vi "ModbusComap.vi"(0 "address":string="192.168.1.205", 1 "port (502)":u16=502, 2 "Unit ID":u8, 3 "Error In":errorcluster) -> (7 "Gen Data":T1 {"TotalFuel(L)" format="%.2f"; "FuelRate(L/H)" format="%.2f"; "ApparentPower(VA)" format="%.2f"; "BattVoltage(V)" format="%.2f"; "Freq(Hz)" format="%.2f"; "RunHours(hr)" format="%.2f"; "PowerFactor" format="%.2f"; "ReactivePower(VAR)" format="%.2f"; "ActivePower(W)" format="%.2f"}, 10 "Error Out":errorcluster)   [LabVIEW 2014]
uses:
  Controls/Gen Data.ctl
  Controls/ModbusState.ctl
  <vilib>/Modbus/master/Modbus Master.lvclass
  <vilib>/Modbus/subvis/Modbus API/Modbus API.lvclass/Modbus API.ctl
  <vilib>/Modbus/subvis/Transmission Data Unit (ADU)/Transmission Data Unit/Transmission Data Unit.lvclass/Transmission Data Unit.ctl
  <vilib>/Modbus/master/Data Access/Unit ID/Set Unit ID Property.vi
  <vilib>/Modbus/subvis/Transmission Data Unit (ADU)/Transmission Data Unit/Data Access/Unit ID/Write Unit ID.vi
  <vilib>/Modbus/subvis/Modbus API/Read Transmission Data Unit.vi
  <vilib>/Modbus/subvis/Modbus API/Write Transmission Data Unit.vi
  <vilib>/Modbus/master/Create Master Instance (TCP).vi
  <vilib>/Modbus/subvis/Transmission Data Unit (ADU)/Transmission Data Unit/Transmission Data Unit.lvclass
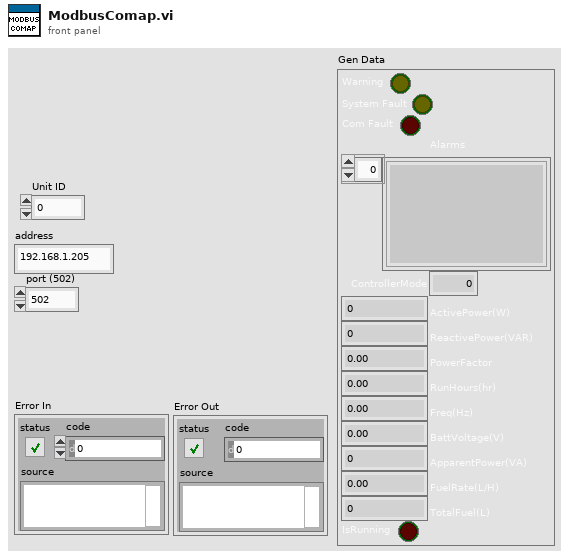
[diagram p1: front panel]
types:
  T1 = typedef "Gen Data.ctl" = cluster{"Warning":bool, "System Fault":bool, "Com Fault":bool, "Alarms":string[], "ControllerMode":u16, "ActivePower(W)":i32, "ReactivePower(VAR)":i32, "PowerFactor":dbl, "RunHours(hr)":dbl, "Freq(Hz)":dbl, "BattVoltage(V)":dbl, "ApparentPower(VA)":i32, "FuelRate(L/H)":dbl, "TotalFuel(L)":u32, "IsRunning":bool}
  T2 = typedef "ModbusState.ctl" = enum16{"Connect", "Disconnect", "Set Basic Objects", "Get Basic Objects", "Read", "Write", "Read/Write"}
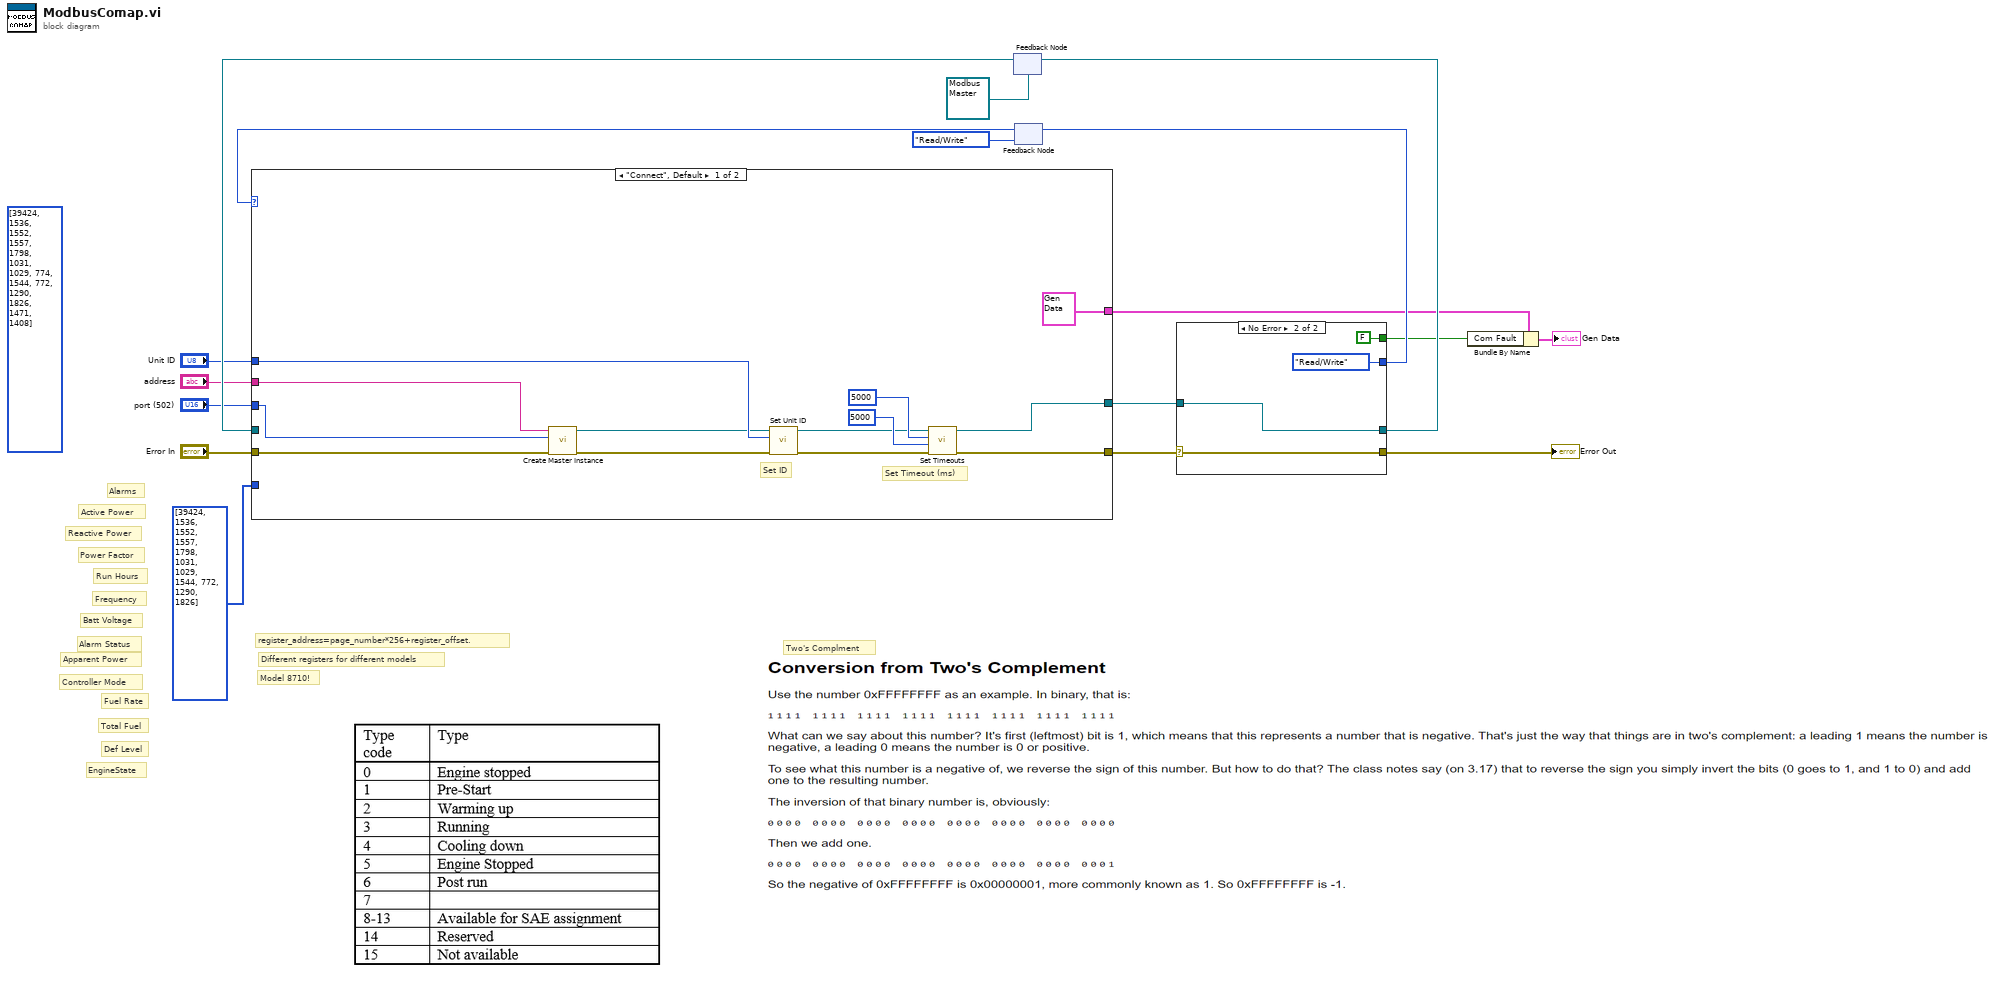
[diagram p0: block diagram]
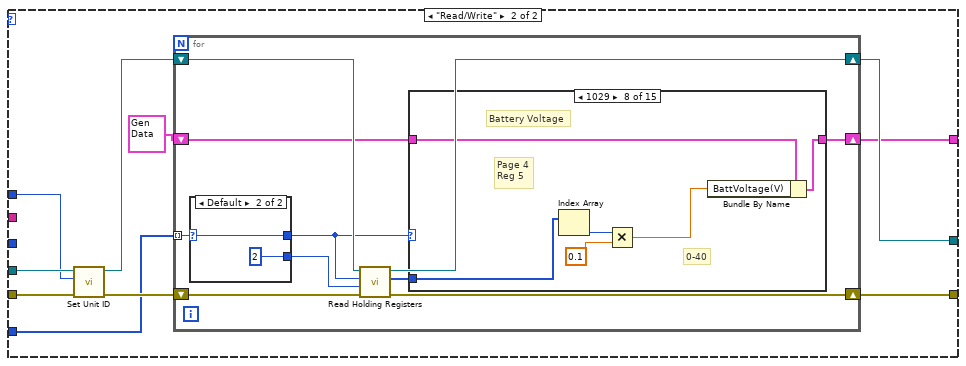
[diagram p2: hidden frame]
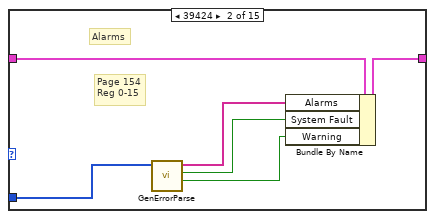
[diagram p4: hidden frame]
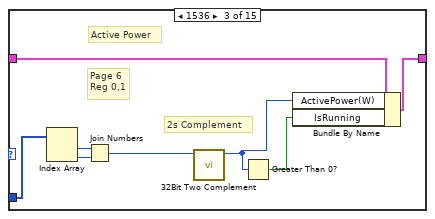
[diagram p5: hidden frame]
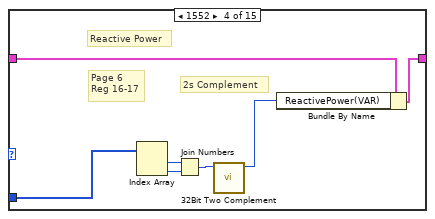
[diagram p6: hidden frame]
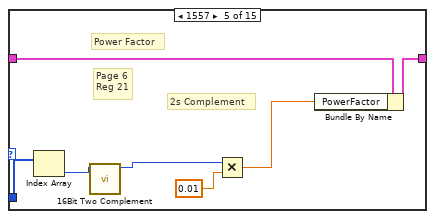
[diagram p7: hidden frame]
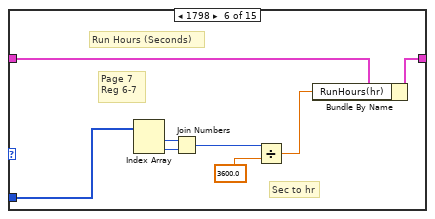
[diagram p8: hidden frame]
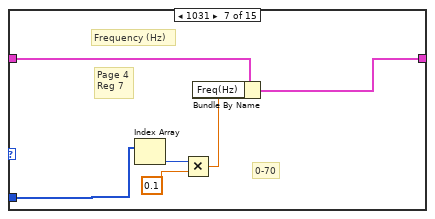
[diagram p9: hidden frame]
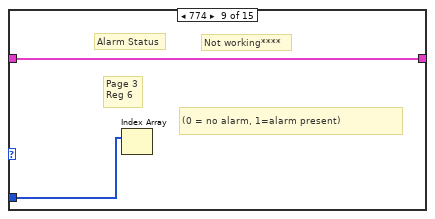
[diagram p10: hidden frame]
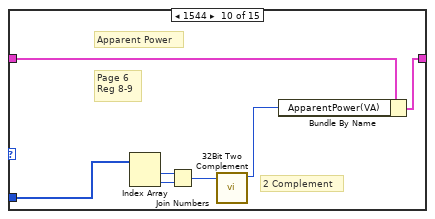
[diagram p11: hidden frame]
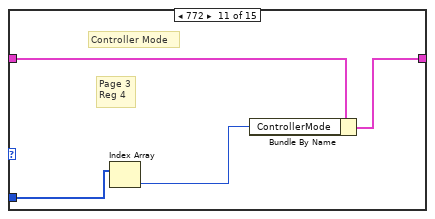
[diagram p12: hidden frame]
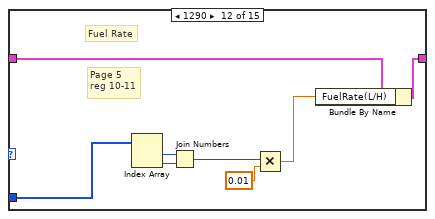
[diagram p13: hidden frame]
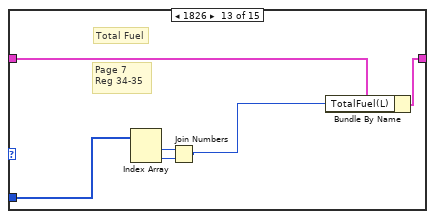
[diagram p14: hidden frame]
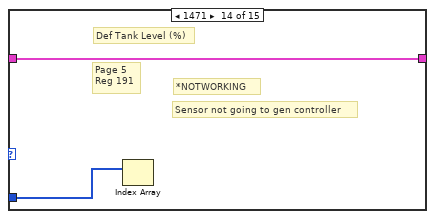
[diagram p15: hidden frame]
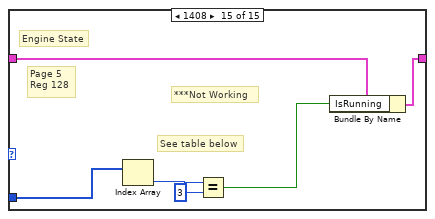
[diagram p16: hidden frame]
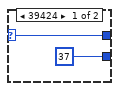
[diagram p17: hidden frame]
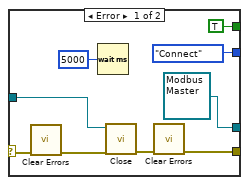
[diagram p18: hidden frame]
diagram:
  (unwired) u16[] [39424, 1536, 1552, 1557, 1798, 1031, 1029, 774, 1544, 772, 1290, 1826, 1471, 1408] ("subarray")
  # "EngineState"
  # "Two's Complment"
  # "Different registers for different models"
  # "Model 8710!"
  # "Def Level"
  # "Alarm Status"
  # "Controller Mode"
  # "register_address=page_number*256+register_offset."
  # "Total Fuel"
  # "Fuel Rate"
  # "Apparent Power"
  # "Run Hours"
  # "Power Factor"
  # "Reactive Power"
  # "Active Power"
  # "Alarms"
  # "Batt Voltage"
  # "Frequency"
  n1 = feedback #1(refnum<class "Modbus Master.lvclass"> refnum ("Modbus master out")) -> (w13:refnum<class "Modbus Master.lvclass">)
  n2 = feedback #2(ModbusState."Read/Write" ("Modbus State In")) -> (w16:T2)
  n3 = case shown="\"Connect\", Default" w16 {
    tunnel: "Error In" -> [w30 w40]
    tunnel: w13 -> [_ w39]
    tunnel: [w19 w35] -> w10
    tunnel: [w18 w36] -> w8
    tunnel: [T1 {"Warning"=FALSE, "System Fault"=FALSE, "Com Fault"=FALSE, "Alarms"=[], "ControllerMode"=0, "ActivePower(W)"=0, "ReactivePower(VAR)"=0, "PowerFactor"=0.0, "RunHours(hr)"=0.0, "Freq(Hz)"=0.0, "BattVoltage(V)"=0.0, "ApparentPower(VA)"=0, "FuelRate(L/H)"=0.0, "TotalFuel(L)"=0, "IsRunning"=FALSE} ("Gen Data") w31] -> w2
    tunnel: "address" -> [w27 _]
    tunnel: "port (502)" -> [w26 _]
    tunnel: "Unit ID" -> [w21 w38]
    tunnel: u16[] [39424, 1536, 1552, 1557, 1798, 1031, 1029, 1544, 772, 1290, 1826] ("subarray") -> [_ w32]
    frame "Connect", Default {
      # "Set Timeout (ms)"
      # "Set ID"
      n4 = call-poly <vilib>:"Create Master Instance.vi"("error in (no error)"=w30, "port (502)"=w26, "address"=w27) -> ("error out"=w24:errorcluster, "TCP master instance"=w20:refnum<class "Modbus Master.lvclass">)  [unwired: 7 in]
      n5 = call <vilib>:"Set Unit ID.vi"("error in (no error)"=w24, "unit ID"=w21, "Modbus master in"=w20) -> ("error out"=w23:errorcluster, "Modbus master out"=w22:refnum<class "Modbus Master.lvclass">)  [unwired: 7 in]
      n6 = call <vilib>:"Set Timeouts.vi"("error in (no error)"=w23, "write operation timeout (ms)"=5000 ("write operation timeout"), "read operation timeout (ms)"=5000 ("read operation timeout"), "Modbus master in"=w22) -> ("error out"=w19:errorcluster, "Modbus master out"=w18:refnum<class "Modbus Master.lvclass">)  [unwired: 6 in]
    }
    frame "Read/Write" {
      n7 = call <vilib>:"Set Unit ID.vi"("error in (no error)"=w40, "unit ID"=w38, "Modbus master in"=w39) -> ("error out"=w33:errorcluster, "Modbus master out"=w34:refnum<class "Modbus Master.lvclass">)  [unwired: 7 in]
      n8 = for {
        tunnel: w32 -> [w50] mode=indexing
        shift-right: [w41] -> w35
        shift-left: w33 -> [w48]
        shift-right: [w46] -> w36
        shift-left: w34 -> [w47]
        shift-right: [w42] -> w31
        shift-left: T1 {"Warning"=FALSE, "System Fault"=FALSE, "Com Fault"=FALSE, "Alarms"=[], "ControllerMode"=0, "ActivePower(W)"=0, "ReactivePower(VAR)"=0, "PowerFactor"=0.0, "RunHours(hr)"=0.0, "Freq(Hz)"=0.0, "BattVoltage(V)"=0.0, "ApparentPower(VA)"=0, "FuelRate(L/H)"=0.0, "TotalFuel(L)"=0, "IsRunning"=FALSE} ("Gen Data") -> [w43]
        n9 = case shown="Default" w50 {
          selector: w50 -> [w135 w138]
          tunnel: [w135 w138] -> w45
          tunnel: [u16 37 ("number of inputs") u16 2 ("number of inputs")] -> w49
          frame 39424 {
          }
          frame Default {
          }
        }
        n10 = call-dynamic "Read Holding Registers.vi"("error in (no error)"=w48, "number of holding registers"=w49, "starting address"=w45, "Modbus master in"=w47) -> ("error out"=w41:errorcluster, "register values"=w44:u16[], "Modbus master out"=w46:refnum<class "Modbus Master.lvclass">)  [unwired: 5 in]
        n11 = case shown="1029" w45 {
          tunnel: w44 -> [_ w55 w63 w68 w77 w83 w91 w95 w101 w104 w112 w117 w122 w128 w132]
          tunnel: w43 -> [w51 w57 w65 w72 w79 w87 w93 w99 w100 w108 w111 w120 w126 w127 w134]
          tunnel: [w51 w56 w64 w71 w78 w86 w92 w98 w100 w107 w110 w119 w125 w127 w133] -> w42
          frame Default {
          }
          frame 39424 {
            # "Page 154\nReg 0-15"
            # "Alarms"
            n12 = call "GenErrorParse.vi"("register values"=w55) -> ("Warning"=w52:bool, "SystemFault"=w53:bool, "Alarms"=w54:string[])  [unwired: 8 in]
            n13 = Bundle By Name(cluster=w57, "Alarms"=w54, "System Fault"=w53, "Warning"=w52) -> (w56:T1)
          }
          frame 1536 {
            # "2s Complement"
            # "Page 6\nReg 0,1"
            # "Active Power"
            n14 = Index Array(array=w63) -> (element #1=w61:u16, element #2=w62:u16)  [unwired: 2 in]
            n15 = Join Numbers(hi=w61, lo=w62) -> ((hi.lo)=w60:u32)
            n16 = call "32Bit Two Complement.vi"("Numeric in"=w60) -> ("Numeric out"=w59:i32)  [unwired: 10 in]
            n17 = Greater Than 0?(x=w59) -> (x > 0?=w58:bool)
            n18 = Bundle By Name(cluster=w65, "ActivePower(W)"=w59, "IsRunning"=w58) -> (w64:T1)
          }
          frame 1552 {
            # "2s Complement"
            # "Page 6\nReg 16-17"
            # "Reactive Power"
            n19 = Index Array(array=w68) -> (element #1=w69:u16, element #2=w70:u16)  [unwired: 2 in]
            n20 = Join Numbers(hi=w69, lo=w70) -> ((hi.lo)=w67:u32)
            n21 = call "32Bit Two Complement.vi"("Numeric in"=w67) -> ("Numeric out"=w66:i32)  [unwired: 10 in]
            n22 = Bundle By Name(cluster=w72, "ReactivePower(VAR)"=w66) -> (w71:T1)
          }
          frame 1557 {
            # "2s Complement"
            # "Page 6\nReg 21"
            # "Power Factor"
            n23 = Index Array(array=w77) -> (element=w74:u16)  [unwired: 1 in]
            n24 = call "16Bit Two Complement.vi"("Numeric in"=w74) -> ("Numeric out"=w73:i16)  [unwired: 10 in]
            n25 = Multiply(x=w73, y=0.01) -> (x*y=w75:dbl)
            n26 = Bundle By Name(cluster=w79, "PowerFactor"=w75) -> (w78:T1)
          }
          frame 1798 {
            # "Sec to hr"
            # "Page 7\nReg 6-7"
            # "Run Hours (Seconds)"
            n27 = Index Array(array=w83) -> (element #1=w84:u16, element #2=w85:u16)  [unwired: 2 in]
            n28 = Join Numbers(hi=w84, lo=w85) -> ((hi.lo)=w80:u32)
            n29 = Divide(x=w80, y=3600.0) -> (x/y=w81:dbl)
            n30 = Bundle By Name(cluster=w87, "RunHours(hr)"=w81) -> (w86:T1)
          }
          frame 1031 {
            # "0-70"
            # "Page 4\nReg 7"
            # "Frequency (Hz)"
            n31 = Index Array(array=w91) -> (element=w90:u16)  [unwired: 1 in]
            n32 = Multiply(x=w90, y=0.1) -> (x*y=w88:dbl)
            n33 = Bundle By Name(cluster=w93, "Freq(Hz)"=w88) -> (w92:T1)
          }
          frame 1029 {
            # "0-40"
            # "Page 4\nReg 5"
            # "Battery Voltage"
            n34 = Index Array(array=w95) -> (element=w97:u16)  [unwired: 1 in]
            n35 = Multiply(x=w97, y=0.1) -> (x*y=w94:dbl)
            n36 = Bundle By Name(cluster=w99, "BattVoltage(V)"=w94) -> (w98:T1)
          }
          frame 774 {
            # "Not working****"
            # "(0 = no alarm, 1=alarm present)"
            # "Page 3\nReg 6"
            # "Alarm Status"
            n37 = Index Array(array=w101) -> ()  [unwired: 1 in, 1 out]
          }
          frame 1544 {
            # "2 Complement"
            # "Page 6\nReg 8-9"
            # "Apparent Power"
            n38 = Index Array(array=w104) -> (element #1=w105:u16, element #2=w106:u16)  [unwired: 2 in]
            n39 = Join Numbers(hi=w105, lo=w106) -> ((hi.lo)=w103:u32)
            n40 = call "32Bit Two Complement.vi"("Numeric in"=w103) -> ("Numeric out"=w102:i32)  [unwired: 10 in]
            n41 = Bundle By Name(cluster=w108, "ApparentPower(VA)"=w102) -> (w107:T1)
          }
          frame 772 {
            # "Page 3\nReg 4"
            # "Controller Mode"
            n42 = Index Array(array=w112) -> (element=w109:u16)  [unwired: 1 in]
            n43 = Bundle By Name(cluster=w111, "ControllerMode"=w109) -> (w110:T1)
          }
          frame 1290 {
            # "Page 5\nreg 10-11"
            # "Fuel Rate"
            n44 = Index Array(array=w117) -> (element #1=w118:u16, element #2=w116:u16)  [unwired: 2 in]
            n45 = Join Numbers(hi=w118, lo=w116) -> ((hi.lo)=w113:u32)
            n46 = Multiply(x=w113, y=0.01) -> (x*y=w114:dbl)
            n47 = Bundle By Name(cluster=w120, "FuelRate(L/H)"=w114) -> (w119:T1)
          }
          frame 1826 {
            # "Page 7\nReg 34-35"
            # "Total Fuel"
            n48 = Index Array(array=w122) -> (element #1=w123:u16, element #2=w124:u16)  [unwired: 2 in]
            n49 = Join Numbers(hi=w123, lo=w124) -> ((hi.lo)=w121:u32)
            n50 = Bundle By Name(cluster=w126, "TotalFuel(L)"=w121) -> (w125:T1)
          }
          frame 1471 {
            # "Sensor not going to gen controller"
            # "*NOTWORKING"
            # "Page 5\nReg 191"
            # "Def Tank Level (%)"
            n51 = Index Array(array=w128) -> ()  [unwired: 1 in, 1 out]
          }
          frame 1408 {
            # "***Not Working"
            # "See table below"
            # "Page 5\nReg 128"
            # "Engine State"
            n52 = Index Array(array=w132) -> (element=w131:u16)  [unwired: 1 in]
            n53 = Equal?(x=w131, y=u16 3) -> (x = y?=w129:bool)
            n54 = Bundle By Name(cluster=w134, "IsRunning"=w129) -> (w133:T1)
          }
        }
      }
    }
  }
  n55 = case shown="No Error" w10 {
    selector: w10 -> [w141 w148]
    tunnel: w8 -> [w145 w151]
    tunnel: [w146 w148] -> w9
    tunnel: [refnum<class "Modbus Master.lvclass"> refnum ("TCP master instance") w151] -> w7
    tunnel: [ModbusState."Connect" ("Modbus State In") ModbusState."Read/Write" ("Modbus State In")] -> w6
    tunnel: [TRUE FALSE] -> w4
    frame Error {
      n56 = call <vilib>:"Clear Errors.vi"("error in (no error)"=w141) -> ("error out"=w140:errorcluster)  [unwired: 5 in, 1 out]
      n57 = Wait (ms)(milliseconds to wait=u32 5000) -> ()  [unwired: 1 out]
      n58 = call-dynamic "Close.vi"("error in (no error)"=w140, "Modbus master in"=w145) -> ("error out"=w147:errorcluster)  [unwired: 9 in]
      n59 = call <vilib>:"Clear Errors.vi"("error in (no error)"=w147) -> ("error out"=w146:errorcluster)  [unwired: 5 in, 1 out]
    }
    frame No Error {
    }
  }
  "Error Out" <- w9
  n60 = feedback-in #1(w7) -> ()
  n61 = feedback-in #2(w6) -> ()
  n62 = Bundle By Name(cluster=w2, "Com Fault"=w4) -> (→"Gen Data":T1)
